vi "JSON File Build String.vi"(7 "1.0? (F)":bool, 8 "error in (no error)":errorcluster, 9 "dsf configuration substring":string, 10 "dsf version substring":string, 11 "version substring":string) -> (0 "error out":errorcluster, 3 "file json string":string)   [LabVIEW 2020, in "DSF Core.lvlib" / "Configuration Session.lvclass"]
uses:
  Configuration Session.lvclass
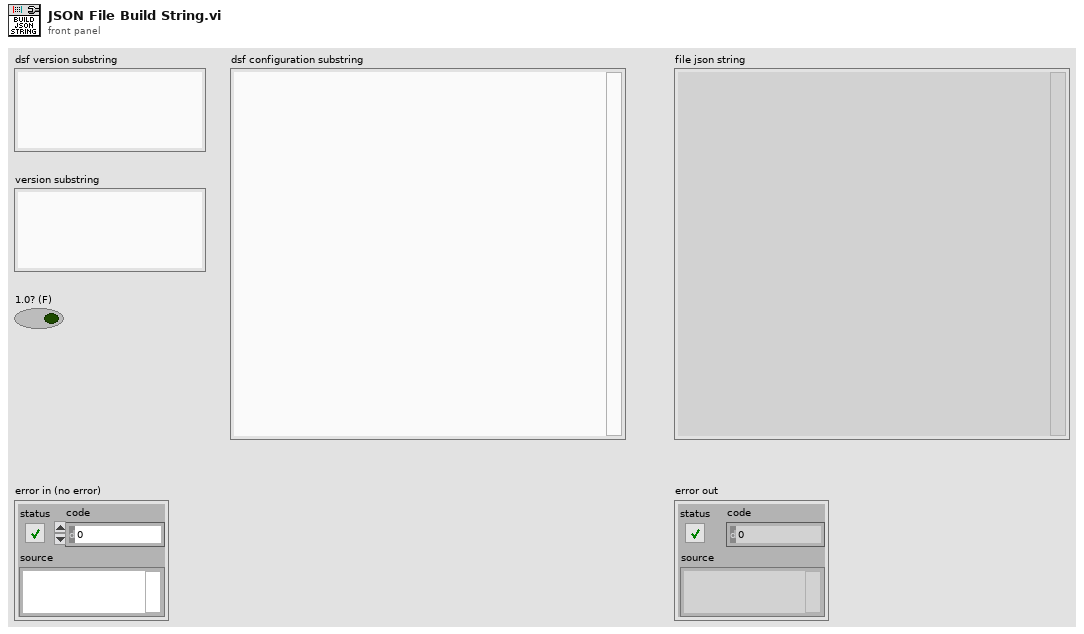
[diagram p1: front panel]
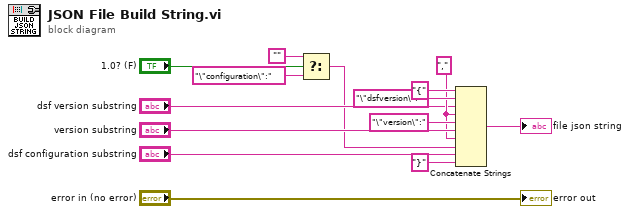
[diagram p0: block diagram]
diagram:
  w9 = "," ("regular expression")
  n1 = Select(t="", s="1.0? (F)", f="\"configuration\":" ("string")) -> (s? t:f=w1:string)
  n2 = Concatenate Strings("{" ("string"), "\"dsfversion\":" ("regular expression"), "dsf version substring", w9, "\"version\":" ("regular expression"), "version substring", w9, w1, "dsf configuration substring", "}" ("string")) -> (→"file json string":string)
  "error out" <- "error in (no error)"
